vi "CUST Poll PDC With Data Waiting.vi"(7 "pollTimeoutMs":i32, 9 "outNumPdcWithData":i32[](array[numeric])=array[4097 elements], 10 "outPseudoPdcIdArr":i32[](array[numeric])=array[4097 elements], 11 "pseudoPdcIdArrayLength":i32) -> (1 "outNumPdcWithData out":i32[](array[numeric]), 2 "outPseudoPdcIdArr out":i32[](array[numeric]), 3 "function return":i32)   [LabVIEW 2013, in "C37118-DLL.lvlib"]
doc: "STRONGRIDIEEEC37118DLL_API int __cdecl pollPdcWithDataWaiting( int pseudoPdcIdArrayLength, int32_t* outPseudoPdcIdArr, int32_t* outNumPdcWithData, int pollTimeoutMs );"
uses:
  C37118-DLL.lvlib
  builds/StrongridDLL/StrongridDLL.dll
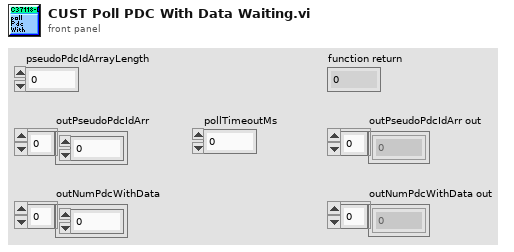
[diagram p1: front panel]
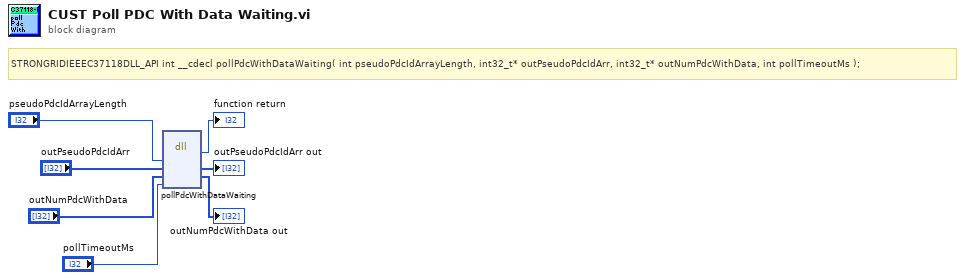
[diagram p0: block diagram]
diagram:
  # "STRONGRIDIEEEC37118DLL_API int __cdecl pollPdcWithDataWaiting( int pseudoPdcIdArrayLength, int32_t* outPseudoPdcIdArr, int32_t* outNumPdcWithData, int pollTimeoutMs );"
  n1 = dll-call lib="C:/dev/OSS/S3DK/builds/StrongridDLL/StrongridDLL.*" fn="pollPdcWithDataWaiting"("pseudoPdcIdArrayLength"="pseudoPdcIdArrayLength", "outPseudoPdcIdArr"="outPseudoPdcIdArr", "outNumPdcWithData"="outNumPdcWithData", "pollTimeoutMs"="pollTimeoutMs") -> ("return type"=→"function return":i32, "outPseudoPdcIdArr"=→"outPseudoPdcIdArr out":i32[], "outNumPdcWithData"=→"outNumPdcWithData out":i32[])  [unwired: 5 in, 2 out]
